vi "(C2K_ADC)_Global.vi"() -> ()   [LabVIEW 2019]
panel:
  in  "File":string="Basic_Config.txt"
  in  "Path":path=path "D:/Projects/C2000/Back_Log/ADC_Step_Responce/Labview/Configuration"
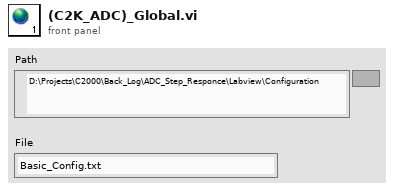
[diagram p1: front panel]
diagram:
